vi "Generate Cooling Data.vi"(9 "i":i32, 11 "Cooling Parameters":cluster{"dt":dbl, "T0":dbl, "Tf":dbl, "k":dbl}) -> (3 "Data":T1)   [LabVIEW 2011]
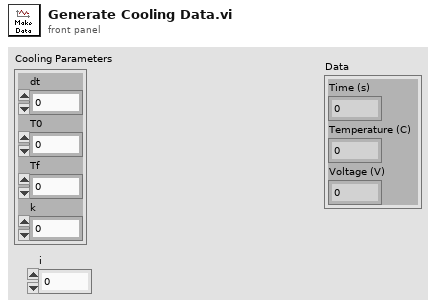
[diagram p1: front panel]
types:
  T1 = cluster{"Time (s)":dbl, "Temperature (C)":dbl, "Voltage (V)":dbl}
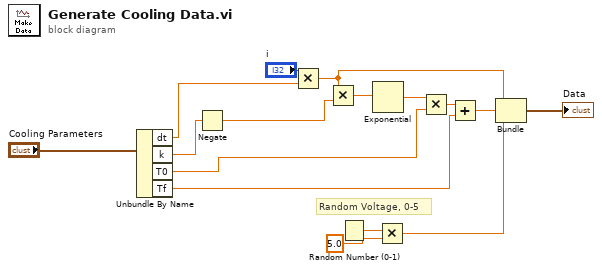
[diagram p0: block diagram]
diagram:
  # "Random Voltage, 0-5"
  n1 = Unbundle By Name("Cooling Parameters") -> ("dt"=w6:dbl, "k"=w5:dbl, "T0"=w2:dbl, "Tf"=w3:dbl)
  n2 = Negate(x=w5) -> (-x=w1:dbl)
  n3 = Multiply(x="i", y=w6) -> (x*y=w4:dbl)
  n4 = Multiply(x=w4, y=w1) -> (x*y=w9:dbl)
  n5 = Random Number (0-1)() -> (number: 0 to 1=w12:dbl)
  n6 = Exponential(1:w9) -> (0:w10:dbl)
  n7 = Multiply(x=w12, y=5.0) -> (x*y=w15:dbl)
  n8 = Multiply(x=w10, y=w2) -> (x*y=w11:dbl)
  n9 = Add(x=w11, y=w3) -> (x+y=w14:dbl)
  n10 = Bundle(w4, w14, w15) -> (→"Data":cluster{dbl, dbl, dbl})  [unwired: 1 in]
